vi "Create Timing Source.vi"(8 "error in (no error)":errorcluster, 11 "TimerDRV in":refnum<class "TimerDRV.lvclass">) -> (0 "error out":errorcluster, 3 "TimerDRV out":refnum<class "TimerDRV.lvclass">)   [LabVIEW 2019, in "TimingDRV Engine.lvlib" / "TimerDRV.lvclass"]
uses:
  TimerDRV.lvclass
  TimerDRV.lvclass/TimerDRV.ctl
  <vilib>/Platform/TimedLoop/scheduler/LVUserAPI/_suppVIs/Create_1MHz_TSource.vi
  <vilib>/Platform/TimedLoop/scheduler/LVUserAPI/_suppVIs/Create_1kHz_TSource.vi
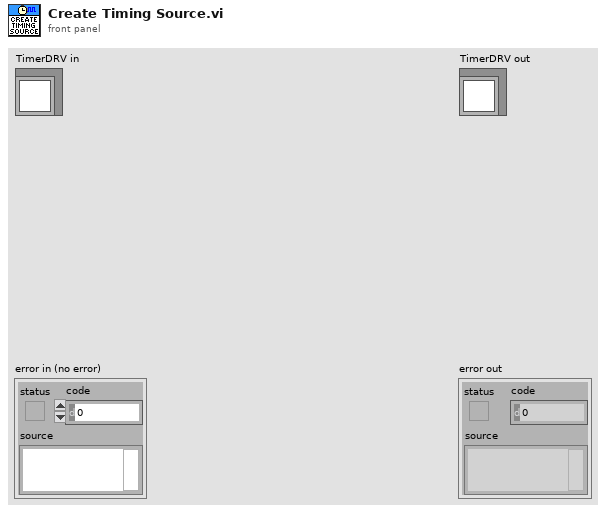
[diagram p1: front panel]
types:
  T1 = typedef "TimingDRV Engine.lvlib/TimerDRV.lvclass/Target Type.ctl" = enum16{"PharLap", "VxWorks", "Windows", "Linux_32_ARM", "Linux_x64"}
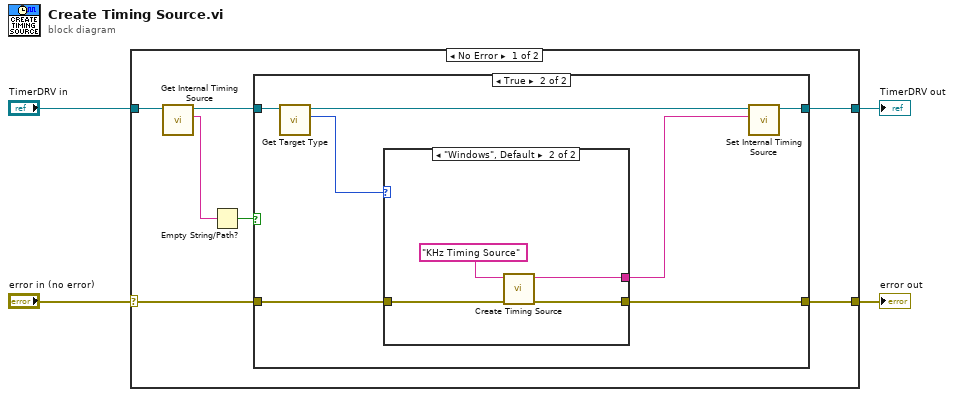
[diagram p0: block diagram]
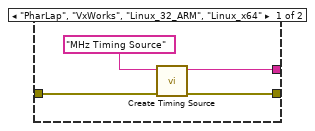
[diagram p3: hidden frame]
diagram:
  n1 = case shown="No Error" "error in (no error)" {
    selector: "error in (no error)" -> [w11 w30]
    tunnel: [w10 w30] -> w3
    tunnel: [w9 w29] -> w1
    tunnel: "TimerDRV in" -> [w8 w29]
    frame No Error {
      n2 = call "Get Internal Timing Source.vi"("TimerDRV in"=w8) -> ("Internal Timing Source"=w6:string, "TimerDRV out"=w7:refnum<class "TimerDRV.lvclass">)  [unwired: 9 in]
      n3 = Empty String/Path?(string/path=w6) -> (empty?=w5:bool)
      n4 = case shown="True" w5 {
        tunnel: w11 -> [w12 w20]
        tunnel: [w12 w17] -> w10
        tunnel: [w13 w15] -> w9
        tunnel: w7 -> [w13 w14]
        frame False {
        }
        frame True {
          n5 = call "Get Target Type.vi"("TimerDRV in"=w14) -> ("Target Type"=w19:T1, "TimerDRV out"=w18:refnum<class "TimerDRV.lvclass">)  [unwired: 9 in]
          n6 = case shown="\"Windows\", Default" w19 {
            tunnel: w20 -> [w23 w28]
            tunnel: [w22 w26] -> w17
            tunnel: [w21 w25] -> w16
            frame "PharLap", "VxWorks", "Linux_32_ARM", "Linux_x64" {
              n7 = call-poly <vilib>:"Create Timing Source.vi"("error in (no error)"=w23, "name (in)"="MHz Timing Source") -> ("error out"=w22:errorcluster, "name (out)"=w21:string)  [unwired: 8 in]
            }
            frame "Windows", Default {
              n8 = call-poly <vilib>:"Create Timing Source.vi"("error in (no error)"=w28, "name (in)"="KHz Timing Source") -> ("error out"=w26:errorcluster, "name (out)"=w25:string)  [unwired: 8 in]
            }
          }
          n9 = call "Set Internal Timing Source.vi"("Internal Timing Source"=w16, "TimerDRV in"=w18) -> ("TimerDRV out"=w15:refnum<class "TimerDRV.lvclass">)  [unwired: 9 in]
        }
      }
    }
    frame Error {
    }
  }
  "error out" <- w3
  "TimerDRV out" <- w1
